vi "Clusterwitharrayvariant.vi"(1 "Cluster In":cluster{"Array In":variant[]}, 2 "String To Append":string, 3 "Base":dbl format="%.2f") -> (0 "Cluster Out":cluster{"Array Out":variant[]})   [LabVIEW 2011]
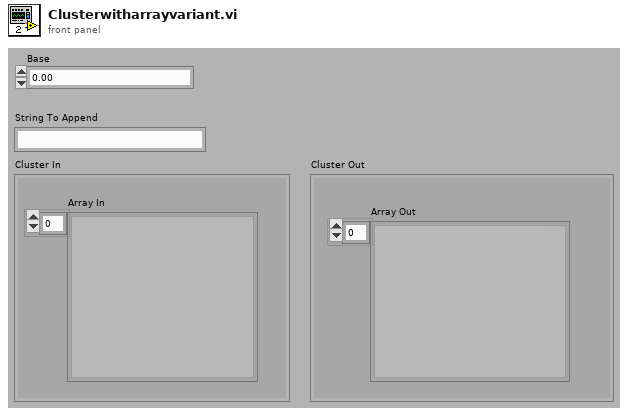
[diagram p1: front panel]
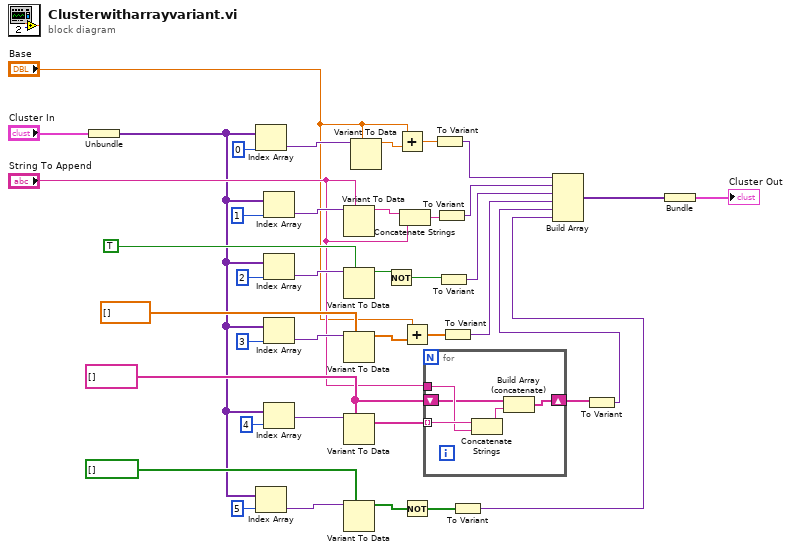
[diagram p0: block diagram]
diagram:
  w14 = string[] []
  n1 = Unbundle("Cluster In") -> ("Array In"=w3:variant[])
  n2 = Index Array(array=w3, index=0) -> (element=w39:variant)
  n3 = Index Array(array=w3, index=5) -> (element=w11:variant)
  n4 = Index Array(array=w3, index=1) -> (element=w34:variant)
  n5 = Index Array(array=w3, index=2) -> (element=w29:variant)
  n6 = Index Array(array=w3, index=3) -> (element=w23:variant)
  n7 = Index Array(array=w3, index=4) -> (element=w16:variant)
  n8 = Variant To Data(type="String To Append", Variant=w34) -> (data=w33:string)  [unwired: 1 in, 1 out]
  n9 = Variant To Data(type=TRUE, Variant=w29) -> (data=w27:bool)  [unwired: 1 in, 1 out]
  n10 = Variant To Data(type=dbl[] [], Variant=w23) -> (data=w21:dbl[])  [unwired: 1 in, 1 out]
  n11 = Variant To Data(type=w14, Variant=w16) -> (data=w15:string[])  [unwired: 1 in, 1 out]
  n12 = Variant To Data(type=bool[] [], Variant=w11) -> (data=w9:bool[])  [unwired: 1 in, 1 out]
  n13 = Variant To Data(type="Base", Variant=w39) -> (data=w38:dbl)  [unwired: 1 in, 1 out]
  n14 = Not(x=w27) -> (.not. x?=w26:bool)
  n15 = Add(x="Base", y=w38) -> (x+y=w37:dbl)
  n16 = Concatenate Strings(w33, "String To Append") -> (w32:string)
  n17 = Add(x="Base", y=w21) -> (x+y=w20:dbl[])
  n18 = Not(x=w9) -> (.not. x?=w8:bool[])
  n19 = for {
    tunnel: w15 -> [w45] mode=indexing
    shift-right: [w41] -> w13
    shift-left: w14 -> [w42]
    tunnel: "String To Append" -> [w44]
    n20 = Concatenate Strings(w45, w44) -> (w43:string)
    n21 = Build Array (concatenate)(w42, w43) -> (w41:string[])
  }
  n22 = To Variant(anything=w37) -> (Variant=w36:variant)
  n23 = To Variant(anything=w32) -> (Variant=w31:variant)
  n24 = To Variant(anything=w26) -> (Variant=w25:variant)
  n25 = To Variant(anything=w20) -> (Variant=w19:variant)
  n26 = To Variant(anything=w8) -> (Variant=w7:variant)
  n27 = To Variant(anything=w13) -> (Variant=w12:variant)
  n28 = Build Array(w36, w31, w25, w19, w12, w7) -> (w2:variant[])
  n29 = Bundle(w2) -> (→"Cluster Out":cluster{variant[]})  [unwired: 1 in]
